vi "Test Snake Moves Vertically.vi"(8 "error in (no error)":errorcluster, 11 "Test Case In":refnum<class "Snake Test.lvclass">) -> (0 "error out":errorcluster, 3 "Test Case Out":refnum<class "Snake Test.lvclass">)   [LabVIEW 2020, in "Snake Test.lvclass"]
uses:
  Snake Test.lvclass
  Snake Test.lvclass/Snake Test.ctl
  source/Snake/Snake.lvclass
  source/Particle/Position.ctl
  source/Particle.lvclass
  <vilib>/Astemes/LUnit/Test Case.lvclass
  C:/Program Files (x86)/National Instruments/LabVIEW 2020/vi.lib/Astemes/LUnit/Test Case.lvclass
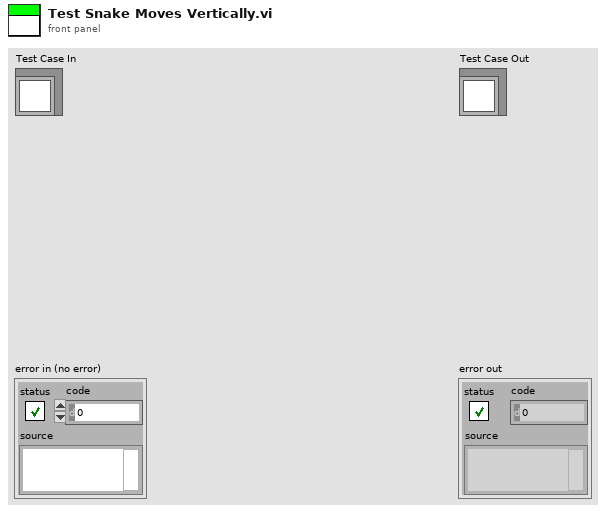
[diagram p1: front panel]
types:
  T1 = typedef "Particle.lvclass/Position.ctl" = cluster{"X":i32, "Y":i32}
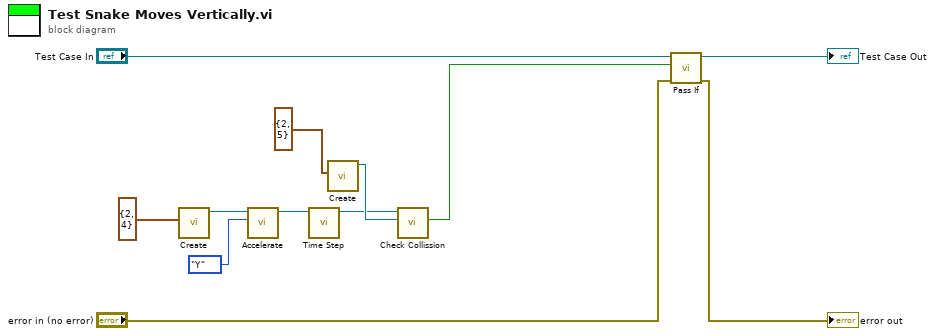
[diagram p0: block diagram]
diagram:
  n1 = call "Create.vi"("Position"=T1 {"X"=2, "Y"=4}) -> ("Snake out"=w8:refnum<class "Snake.lvclass">)  [unwired: 10 in]
  n2 = call "Accelerate.vi"("Direction"=enum16{"X", "-X", "Y", "-Y"}."Y", "Snake in"=w8) -> ("Snake out"=w2:refnum<class "Snake.lvclass">)  [unwired: 9 in]
  n3 = call "Time Step.vi"("Snake in"=w2) -> ("Snake out"=w1:refnum<class "Snake.lvclass">)  [unwired: 10 in]
  n4 = call "Create.vi"("Position"=T1 {"X"=2, "Y"=5}) -> ("Particle out"=w6:refnum<class "Particle.lvclass">)  [unwired: 10 in]
  n5 = call "Check Collission.vi"("Particle"=w6, "Snake in"=w1) -> ("Collided?"=w5:bool)  [unwired: 8 in, 1 out]
  n6 = call <vilib>:"Pass If.vi"("error in (no error)"="error in (no error)", "Pass?"=w5, "LUnit Test Case In"="Test Case In") -> ("error out"=→"error out":errorcluster, "LUnit Test Case Out"=→"Test Case Out":refnum<class "Snake Test.lvclass">)  [unwired: 7 in]
